vi "Actor Core.vi"(8 "error in (no error)":errorcluster, 11 "Parrot in":refnum<class "Parrot.lvclass">) -> (0 "error out":errorcluster, 3 "Parrot out":refnum<class "Parrot.lvclass">)   [LabVIEW 2016, in "Parrot.lvclass"]
doc: "--\nCopyright © 2017 Composed SystemsI All rights reserved.\n\nAuthor: Jon McBee <jon.mcbee@composed.io>\n\nThis library is provided \"AS IS\" ,WITHOUT WARRANTIES OR\nCONDITIONS OF ANY KIND, either express or implied.\n\nComposed Systems -- composed.io\n\nStream 0.0.1.1\nJon McBee - Composed Systems\nCopyright (c) 2017, Composed Systems"
uses:
  <userlib>/Composed Systems/Stream/Sandbox/Async Actor Test/Parrot Actor/Parrot.lvclass
  D:/Repos/Stream/software/Mediator/Classes/Mediated Actor/Mediated Actor.lvclass
  <userlib>/Composed Systems/Stream/Sandbox/Async Actor Test/Parrot Actor/Parrot.lvclass/Parrot.ctl
  <userlib>/Composed Systems/Stream/Mediator/Classes/Message Broker Interface/Message Broker Interface.lvclass
  <userlib>/Composed Systems/Stream/Mediator/Classes/Mediated Asynchronous Actor/Mediated Asynchronous Actor.lvclass
  <userlib>/Composed Systems/Stream/Mediator/Classes/Mediated Actor/Mediated Actor.lvclass
panel:
  out "Received String":string
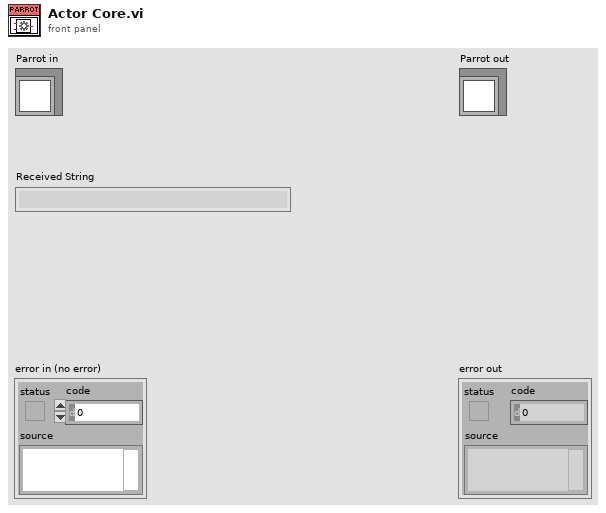
[diagram p1: front panel]
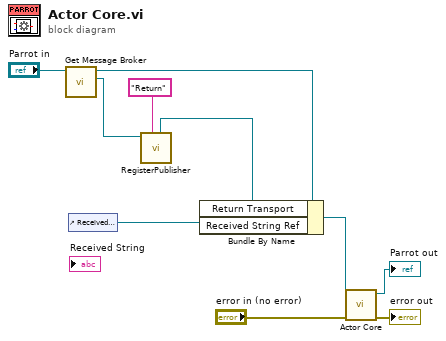
[diagram p0: block diagram]
diagram:
  n1 = call <userlib>:"Get Message Broker.vi"("Mediated Actor in"="Parrot in") -> ("Message Broker"=w3:refnum<class "Message Broker Interface.lvclass">, "Mediated Actor out"=w4:refnum<class "Parrot.lvclass">)  [unwired: 9 in]
  n2 = control-ref of="Received String"() -> (w6:refnum<vi>)
  n3 = call-dynamic "RegisterPublisher.vi"("Topic Name"="Return", "Message Broker Interface in"=w3) -> ("Transport"=w1:refnum<class "Message Transport Queue.lvclass">)  [unwired: 5 in, 4 out]
  n4 = Bundle By Name(cluster=w4, "Return Transport"=w1, "Received String Ref"=w6) -> (w7:refnum<class "Parrot.lvclass">)
  n5 = call-parent "Actor Core.vi"("error in (no error)"="error in (no error)", "Mediated Asynchronous Actor in"=w7) -> ("error out"=→"error out":errorcluster, "Mediated Asynchronous Actor out"=→"Parrot out":refnum<class "Parrot.lvclass">)  [unwired: 8 in]
